vi "Teleop.vi"(10 "Match Info":T1={"Autonomous Elapsed Seconds"=0.0, "TeleOp Elapsed Seconds"=0.0, "Disabled Elapsed Seconds"=0.0, "Visited Autonomous"=FALSE, "Visited TeleOp"=FALSE, "Visited Disabled"=FALSE, "Autonomous Settings"={"Autonomous Style"=enum."Independent", "VI Refnum"=refnum}}, 11 "Call Context":T2) -> ()   [LabVIEW 2013]
doc: "This VI is called for each TeleOp packet received from the DS where the robot is not disabled. It is often used to read from the joysticks and update I/O or to update setpoints for timed control loops. It should complete and return within 20 milliseconds or it may miss DS packets."
uses:
  <vilib>/Rock Robotics/WPI/DriverStation/WPI_DriverStationDerivedRobotMode.ctl
  <vilib>/Rock Robotics/WPI/DriverStation/WPI_DriverStationMatch Info.ctl
  Robot Global Data.vi
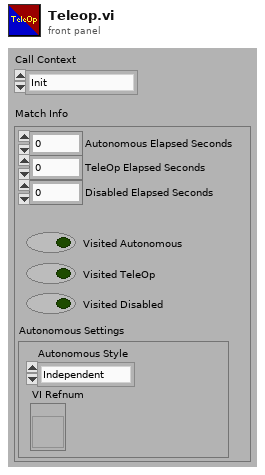
[diagram p1: front panel]
types:
  T1 = typedef "WPI_DriverStationMatch Info.ctl" = cluster{"Autonomous Elapsed Seconds":dbl, "TeleOp Elapsed Seconds":dbl, "Disabled Elapsed Seconds":dbl, "Visited Autonomous":bool, "Visited TeleOp":bool, "Visited Disabled":bool, "Autonomous Settings":cluster{"Autonomous Style":enum16{"Iterative", "Independent"}, "VI Refnum":refnum<vi>}}
  T2 = typedef "WPI_DriverStationDerivedRobotMode.ctl" = enum16{"Init", "Execute", "Stop"}
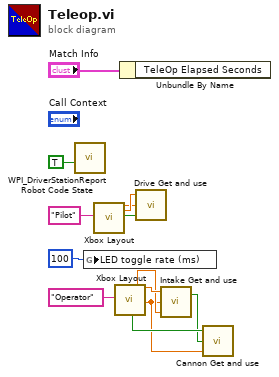
[diagram p0: block diagram]
diagram:
  n1 = call <vilib>:"WPI_DriverStationReport Robot Code State.vi"("TeleOp"=TRUE ("Autonomous")) -> ()  [unwired: 10 in, 1 out]
  n2 = global write "Robot Global Data.vi" "LED toggle rate (ms)"(u32 100 ("LED ms toggle rate")) -> ()
  n3 = call "Xbox Layout.vi"("Joystick Name"="Pilot" ("refnum name")) -> ("Left Stick Y"=w5:dbl, "Left Stick X"=w6:dbl, "Left Stick Touch"=w4:bool)  [unwired: 3 in, 13 out]
  n4 = call "Xbox Layout.vi"("Joystick Name"="Operator" ("refnum name")) -> ("X"=w9:bool, "L+R Throttles"=w7:dbl, "Left Stick Y"=w8:dbl, "Right Stick Y"=w1:dbl)  [unwired: 3 in, 12 out]
  n5 = Unbundle By Name("Match Info") -> ()  [unwired: 1 out]
  n6 = call "Drive Get and use.vi"("Slow Drive"=w4, "Y - Axis"=w5, "X - Axis"=w6) -> ()
  n7 = call "Intake Get and use.vi"("TakeBall"=w7, "Cannon vbus"=w1, "Upper Claw"=w8) -> ("InTake Max"=w3:bool)  [unwired: 1 out]
  n8 = call "Cannon Get and use.vi"("Move"=w1, "InTake Max"=w3, "Fire"=w9) -> ()  [unwired: 1 out]
